vi "support.read_and_free_string_at_address.vi"(8 "error in (no error)":errorcluster, 11 "string_ptr":u64) -> (0 "error out":errorcluster, 3 "string":string)   [LabVIEW 2020, in "toml_edit.lvlib"]
uses:
  toml_edit.lvlib
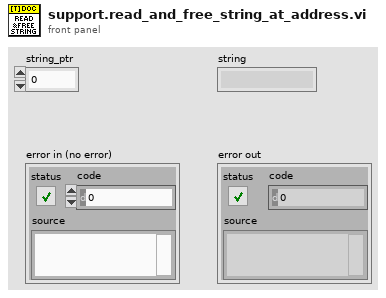
[diagram p1: front panel]
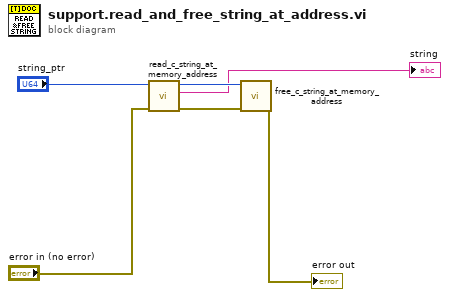
[diagram p0: block diagram]
diagram:
  n1 = call "read_c_string_at_memory_address.vi"("error in (no error)"="error in (no error)", "memory_address"="string_ptr") -> ("error out"=w5:errorcluster, "string"=→"string":string, "memory_address out"=w4:u64)  [unwired: 7 in]
  n2 = call "free_c_string_at_memory_address.vi"("error in (no error)"=w5, "memory_address"=w4) -> ("error out"=→"error out":errorcluster)  [unwired: 9 in]
